vi "Main.vi"() -> ()   [LabVIEW 2021] (continued)
                    w601 = T9 9 items=["刷新间隔", "波特率", "布尔1设置项", "布尔2设置项", "布尔3设置项", "布尔4设置项", "布尔5设置项", "布尔6设置项", "布尔7设置项", "布尔8设置项", "显控1设置", "显控2设置", "显控3设置", "显控4设置", "显控5设置", "显控6设置", "显控7设置", "显控8设置", "显控9设置", "显控10设置", "显控11设置", "显控12设置", "设控1设置", "设控2设置", "设控3设置", "设控4设置", "设控5设置", "设控6设置", "设控7设置", "设控8设置", "曲线1设置", "曲线2设置", "曲线3设置", "曲线4设置", "曲线5设置", "曲线6设置", "曲线7设置", "曲线8设置", "曲线9设置", "曲线10设置", "曲线11设置", "曲线12设置", "曲线13设置", "曲线14设置", "曲线15设置", "曲线16设置", "曲线17设置", "曲线18设置", "曲线19设置", "曲线20设置", "曲线21设置", "曲线22设置", "曲线23设置", "曲线24设置", "曲线25设置", "曲线26设置", "曲线27设置", "曲线28设置", "曲线29设置", "曲线30设置", "曲线31设置", "曲线32设置", "曲线33设置", "曲线34设置", "曲线35设置", "曲线36设置", "曲线37设置", "曲线38设置", "曲线39设置", "曲线40设置", "曲线41设置", "曲线42设置", "曲线43设置", "曲线44设置", "曲线45设置", "曲线46设置", "曲线47设置", "曲线48设置", "曲线49设置", "曲线50设置", "曲线51设置", "曲线52设置", "曲线53设置", "曲线54设置", "曲线55设置", "曲线56设置", "曲线57设置", "曲线58设置", "曲线59设置", "曲线60设置", "曲线61设置", "曲线62设置", "曲线63设置", "曲线64设置", "ID值", "数据模式"] ("DataInitDef")
                    n457 = property on="表格" class="Tbl (严格)"() -> ("Selection Start"=w609:T1)  [unwired: 2 in, 2 out]
                    n458 = Unbundle By Name(w609) -> ("Row"=w608:i32)
                    n459 = property on="表格" class="Tbl (严格)"() -> ("Value"=w610:string[][])  [unwired: 2 in, 2 out]
                    n460 = Number To Decimal String(number=w608) -> (decimal integer string=w611:string)  [unwired: 1 in]
                    n461 = Index Array(array=w610, index (row)=w608, index (col)=0 ("禁用的索引 (列)")) -> (element=w607:string)
                    n462 = String Subset(string=w607, length (rest)=10 ("长度（剩余）")) -> (substring=w606:string)  [unwired: 1 in]
                    n463 = invoke on="控件配置文件" class="Tbl (严格)" method="Set Cell Value"("X Index"=1 ("X索引"), "Y Index"=w601, "Value"=w611) -> ()  [unwired: 3 in, 6 out]
                    n464 = property on="布尔 8" class="Bool (严格)"("Caption.Text"=w606) -> ()  [unwired: 2 in, 2 out]
                    n465 = property on="布控8设置" class="Str"("Val(Sgnl)"=w606) -> ()  [unwired: 2 in, 2 out]
                    n466 = invoke on="控件配置文件" class="Tbl (严格)" method="Set Cell Value"("X Index"=0 ("X索引"), "Y Index"=w601, "Value"=w606) -> ()  [unwired: 3 in, 6 out]
                  }
                  frame "关联到显控1" {
                    w612 = T9 10 items=["刷新间隔", "波特率", "布尔1设置项", "布尔2设置项", "布尔3设置项", "布尔4设置项", "布尔5设置项", "布尔6设置项", "布尔7设置项", "布尔8设置项", "显控1设置", "显控2设置", "显控3设置", "显控4设置", "显控5设置", "显控6设置", "显控7设置", "显控8设置", "显控9设置", "显控10设置", "显控11设置", "显控12设置", "设控1设置", "设控2设置", "设控3设置", "设控4设置", "设控5设置", "设控6设置", "设控7设置", "设控8设置", "曲线1设置", "曲线2设置", "曲线3设置", "曲线4设置", "曲线5设置", "曲线6设置", "曲线7设置", "曲线8设置", "曲线9设置", "曲线10设置", "曲线11设置", "曲线12设置", "曲线13设置", "曲线14设置", "曲线15设置", "曲线16设置", "曲线17设置", "曲线18设置", "曲线19设置", "曲线20设置", "曲线21设置", "曲线22设置", "曲线23设置", "曲线24设置", "曲线25设置", "曲线26设置", "曲线27设置", "曲线28设置", "曲线29设置", "曲线30设置", "曲线31设置", "曲线32设置", "曲线33设置", "曲线34设置", "曲线35设置", "曲线36设置", "曲线37设置", "曲线38设置", "曲线39设置", "曲线40设置", "曲线41设置", "曲线42设置", "曲线43设置", "曲线44设置", "曲线45设置", "曲线46设置", "曲线47设置", "曲线48设置", "曲线49设置", "曲线50设置", "曲线51设置", "曲线52设置", "曲线53设置", "曲线54设置", "曲线55设置", "曲线56设置", "曲线57设置", "曲线58设置", "曲线59设置", "曲线60设置", "曲线61设置", "曲线62设置", "曲线63设置", "曲线64设置", "ID值", "数据模式"] ("DataInitDef")
                    n467 = property on="表格" class="Tbl (严格)"() -> ("Selection Start"=w622:T1)  [unwired: 2 in, 2 out]
                    n468 = Unbundle By Name(w622) -> ("Row"=w619:i32)
                    n469 = property on="表格" class="Tbl (严格)"() -> ("Value"=w621:string[][])  [unwired: 2 in, 2 out]
                    n470 = Number To Decimal String(number=w619) -> (decimal integer string=w616:string)  [unwired: 1 in]
                    n471 = Index Array(array=w621, index (row)=w619, index (col)=0 ("禁用的索引 (列)")) -> (element=w614:string)
                    n472 = String Subset(string=w614, length (rest)=16 ("长度（剩余）")) -> (substring=w613:string)  [unwired: 1 in]
                    n473 = invoke on="控件配置文件" class="Tbl (严格)" method="Set Cell Value"("X Index"=1 ("X索引"), "Y Index"=w612, "Value"=w616) -> ()  [unwired: 3 in, 6 out]
                    n474 = property on="显控1设置" class="Str"("Val(Sgnl)"=w613) -> ()  [unwired: 2 in, 2 out]
                    n475 = property on="显控1" class="Str"("Caption.Text"=w613) -> ()  [unwired: 2 in, 2 out]
                    n476 = invoke on="控件配置文件" class="Tbl (严格)" method="Set Cell Value"("X Index"=0 ("X索引"), "Y Index"=w612, "Value"=w613) -> ()  [unwired: 3 in, 6 out]
                  }
                  frame "关联到显控2" {
                    w623 = T9 11 items=["刷新间隔", "波特率", "布尔1设置项", "布尔2设置项", "布尔3设置项", "布尔4设置项", "布尔5设置项", "布尔6设置项", "布尔7设置项", "布尔8设置项", "显控1设置", "显控2设置", "显控3设置", "显控4设置", "显控5设置", "显控6设置", "显控7设置", "显控8设置", "显控9设置", "显控10设置", "显控11设置", "显控12设置", "设控1设置", "设控2设置", "设控3设置", "设控4设置", "设控5设置", "设控6设置", "设控7设置", "设控8设置", "曲线1设置", "曲线2设置", "曲线3设置", "曲线4设置", "曲线5设置", "曲线6设置", "曲线7设置", "曲线8设置", "曲线9设置", "曲线10设置", "曲线11设置", "曲线12设置", "曲线13设置", "曲线14设置", "曲线15设置", "曲线16设置", "曲线17设置", "曲线18设置", "曲线19设置", "曲线20设置", "曲线21设置", "曲线22设置", "曲线23设置", "曲线24设置", "曲线25设置", "曲线26设置", "曲线27设置", "曲线28设置", "曲线29设置", "曲线30设置", "曲线31设置", "曲线32设置", "曲线33设置", "曲线34设置", "曲线35设置", "曲线36设置", "曲线37设置", "曲线38设置", "曲线39设置", "曲线40设置", "曲线41设置", "曲线42设置", "曲线43设置", "曲线44设置", "曲线45设置", "曲线46设置", "曲线47设置", "曲线48设置", "曲线49设置", "曲线50设置", "曲线51设置", "曲线52设置", "曲线53设置", "曲线54设置", "曲线55设置", "曲线56设置", "曲线57设置", "曲线58设置", "曲线59设置", "曲线60设置", "曲线61设置", "曲线62设置", "曲线63设置", "曲线64设置", "ID值", "数据模式"] ("DataInitDef")
                    n477 = property on="表格" class="Tbl (严格)"() -> ("Selection Start"=w632:T1)  [unwired: 2 in, 2 out]
                    n478 = Unbundle By Name(w632) -> ("Row"=w630:i32)
                    n479 = property on="表格" class="Tbl (严格)"() -> ("Value"=w631:string[][])  [unwired: 2 in, 2 out]
                    n480 = Number To Decimal String(number=w630) -> (decimal integer string=w627:string)  [unwired: 1 in]
                    n481 = Index Array(array=w631, index (row)=w630, index (col)=0 ("禁用的索引 (列)")) -> (element=w625:string)
                    n482 = String Subset(string=w625, length (rest)=16 ("长度（剩余）")) -> (substring=w624:string)  [unwired: 1 in]
                    n483 = invoke on="控件配置文件" class="Tbl (严格)" method="Set Cell Value"("X Index"=1 ("X索引"), "Y Index"=w623, "Value"=w627) -> ()  [unwired: 3 in, 6 out]
                    n484 = property on="显控2设置" class="Str"("Val(Sgnl)"=w624) -> ()  [unwired: 2 in, 2 out]
                    n485 = property on="显控2" class="Str"("Caption.Text"=w624) -> ()  [unwired: 2 in, 2 out]
                    n486 = invoke on="控件配置文件" class="Tbl (严格)" method="Set Cell Value"("X Index"=0 ("X索引"), "Y Index"=w623, "Value"=w624) -> ()  [unwired: 3 in, 6 out]
                  }
                  frame "关联到显控3" {
                    w634 = T9 12 items=["刷新间隔", "波特率", "布尔1设置项", "布尔2设置项", "布尔3设置项", "布尔4设置项", "布尔5设置项", "布尔6设置项", "布尔7设置项", "布尔8设置项", "显控1设置", "显控2设置", "显控3设置", "显控4设置", "显控5设置", "显控6设置", "显控7设置", "显控8设置", "显控9设置", "显控10设置", "显控11设置", "显控12设置", "设控1设置", "设控2设置", "设控3设置", "设控4设置", "设控5设置", "设控6设置", "设控7设置", "设控8设置", "曲线1设置", "曲线2设置", "曲线3设置", "曲线4设置", "曲线5设置", "曲线6设置", "曲线7设置", "曲线8设置", "曲线9设置", "曲线10设置", "曲线11设置", "曲线12设置", "曲线13设置", "曲线14设置", "曲线15设置", "曲线16设置", "曲线17设置", "曲线18设置", "曲线19设置", "曲线20设置", "曲线21设置", "曲线22设置", "曲线23设置", "曲线24设置", "曲线25设置", "曲线26设置", "曲线27设置", "曲线28设置", "曲线29设置", "曲线30设置", "曲线31设置", "曲线32设置", "曲线33设置", "曲线34设置", "曲线35设置", "曲线36设置", "曲线37设置", "曲线38设置", "曲线39设置", "曲线40设置", "曲线41设置", "曲线42设置", "曲线43设置", "曲线44设置", "曲线45设置", "曲线46设置", "曲线47设置", "曲线48设置", "曲线49设置", "曲线50设置", "曲线51设置", "曲线52设置", "曲线53设置", "曲线54设置", "曲线55设置", "曲线56设置", "曲线57设置", "曲线58设置", "曲线59设置", "曲线60设置", "曲线61设置", "曲线62设置", "曲线63设置", "曲线64设置", "ID值", "数据模式"] ("DataInitDef")
                    n487 = property on="表格" class="Tbl (严格)"() -> ("Selection Start"=w643:T1)  [unwired: 2 in, 2 out]
                    n488 = Unbundle By Name(w643) -> ("Row"=w641:i32)
                    n489 = property on="表格" class="Tbl (严格)"() -> ("Value"=w642:string[][])  [unwired: 2 in, 2 out]
                    n490 = Number To Decimal String(number=w641) -> (decimal integer string=w638:string)  [unwired: 1 in]
                    n491 = Index Array(array=w642, index (row)=w641, index (col)=0 ("禁用的索引 (列)")) -> (element=w636:string)
                    n492 = String Subset(string=w636, length (rest)=16 ("长度（剩余）")) -> (substring=w635:string)  [unwired: 1 in]
                    n493 = invoke on="控件配置文件" class="Tbl (严格)" method="Set Cell Value"("X Index"=1 ("X索引"), "Y Index"=w634, "Value"=w638) -> ()  [unwired: 3 in, 6 out]
                    n494 = property on="显控3设置" class="Str"("Val(Sgnl)"=w635) -> ()  [unwired: 2 in, 2 out]
                    n495 = property on="显控3" class="Str"("Caption.Text"=w635) -> ()  [unwired: 2 in, 2 out]
                    n496 = invoke on="控件配置文件" class="Tbl (严格)" method="Set Cell Value"("X Index"=0 ("X索引"), "Y Index"=w634, "Value"=w635) -> ()  [unwired: 3 in, 6 out]
                  }
                  frame "关联到显控4" {
                    w645 = T9 13 items=["刷新间隔", "波特率", "布尔1设置项", "布尔2设置项", "布尔3设置项", "布尔4设置项", "布尔5设置项", "布尔6设置项", "布尔7设置项", "布尔8设置项", "显控1设置", "显控2设置", "显控3设置", "显控4设置", "显控5设置", "显控6设置", "显控7设置", "显控8设置", "显控9设置", "显控10设置", "显控11设置", "显控12设置", "设控1设置", "设控2设置", "设控3设置", "设控4设置", "设控5设置", "设控6设置", "设控7设置", "设控8设置", "曲线1设置", "曲线2设置", "曲线3设置", "曲线4设置", "曲线5设置", "曲线6设置", "曲线7设置", "曲线8设置", "曲线9设置", "曲线10设置", "曲线11设置", "曲线12设置", "曲线13设置", "曲线14设置", "曲线15设置", "曲线16设置", "曲线17设置", "曲线18设置", "曲线19设置", "曲线20设置", "曲线21设置", "曲线22设置", "曲线23设置", "曲线24设置", "曲线25设置", "曲线26设置", "曲线27设置", "曲线28设置", "曲线29设置", "曲线30设置", "曲线31设置", "曲线32设置", "曲线33设置", "曲线34设置", "曲线35设置", "曲线36设置", "曲线37设置", "曲线38设置", "曲线39设置", "曲线40设置", "曲线41设置", "曲线42设置", "曲线43设置", "曲线44设置", "曲线45设置", "曲线46设置", "曲线47设置", "曲线48设置", "曲线49设置", "曲线50设置", "曲线51设置", "曲线52设置", "曲线53设置", "曲线54设置", "曲线55设置", "曲线56设置", "曲线57设置", "曲线58设置", "曲线59设置", "曲线60设置", "曲线61设置", "曲线62设置", "曲线63设置", "曲线64设置", "ID值", "数据模式"] ("DataInitDef")
                    n497 = property on="表格" class="Tbl (严格)"() -> ("Selection Start"=w654:T1)  [unwired: 2 in, 2 out]
                    n498 = Unbundle By Name(w654) -> ("Row"=w652:i32)
                    n499 = property on="表格" class="Tbl (严格)"() -> ("Value"=w653:string[][])  [unwired: 2 in, 2 out]
                    n500 = Number To Decimal String(number=w652) -> (decimal integer string=w649:string)  [unwired: 1 in]
                    n501 = Index Array(array=w653, index (row)=w652, index (col)=0 ("禁用的索引 (列)")) -> (element=w647:string)
                    n502 = String Subset(string=w647, length (rest)=16 ("长度（剩余）")) -> (substring=w646:string)  [unwired: 1 in]
                    n503 = invoke on="控件配置文件" class="Tbl (严格)" method="Set Cell Value"("X Index"=1 ("X索引"), "Y Index"=w645, "Value"=w649) -> ()  [unwired: 3 in, 6 out]
                    n504 = property on="显控4设置" class="Str"("Val(Sgnl)"=w646) -> ()  [unwired: 2 in, 2 out]
                    n505 = property on="显控4" class="Str"("Caption.Text"=w646) -> ()  [unwired: 2 in, 2 out]
                    n506 = invoke on="控件配置文件" class="Tbl (严格)" method="Set Cell Value"("X Index"=0 ("X索引"), "Y Index"=w645, "Value"=w646) -> ()  [unwired: 3 in, 6 out]
                  }
                  frame "关联到显控5" {
                    w656 = T9 14 items=["刷新间隔", "波特率", "布尔1设置项", "布尔2设置项", "布尔3设置项", "布尔4设置项", "布尔5设置项", "布尔6设置项", "布尔7设置项", "布尔8设置项", "显控1设置", "显控2设置", "显控3设置", "显控4设置", "显控5设置", "显控6设置", "显控7设置", "显控8设置", "显控9设置", "显控10设置", "显控11设置", "显控12设置", "设控1设置", "设控2设置", "设控3设置", "设控4设置", "设控5设置", "设控6设置", "设控7设置", "设控8设置", "曲线1设置", "曲线2设置", "曲线3设置", "曲线4设置", "曲线5设置", "曲线6设置", "曲线7设置", "曲线8设置", "曲线9设置", "曲线10设置", "曲线11设置", "曲线12设置", "曲线13设置", "曲线14设置", "曲线15设置", "曲线16设置", "曲线17设置", "曲线18设置", "曲线19设置", "曲线20设置", "曲线21设置", "曲线22设置", "曲线23设置", "曲线24设置", "曲线25设置", "曲线26设置", "曲线27设置", "曲线28设置", "曲线29设置", "曲线30设置", "曲线31设置", "曲线32设置", "曲线33设置", "曲线34设置", "曲线35设置", "曲线36设置", "曲线37设置", "曲线38设置", "曲线39设置", "曲线40设置", "曲线41设置", "曲线42设置", "曲线43设置", "曲线44设置", "曲线45设置", "曲线46设置", "曲线47设置", "曲线48设置", "曲线49设置", "曲线50设置", "曲线51设置", "曲线52设置", "曲线53设置", "曲线54设置", "曲线55设置", "曲线56设置", "曲线57设置", "曲线58设置", "曲线59设置", "曲线60设置", "曲线61设置", "曲线62设置", "曲线63设置", "曲线64设置", "ID值", "数据模式"] ("DataInitDef")
                    n507 = property on="表格" class="Tbl (严格)"() -> ("Selection Start"=w665:T1)  [unwired: 2 in, 2 out]
                    n508 = Unbundle By Name(w665) -> ("Row"=w663:i32)
                    n509 = property on="表格" class="Tbl (严格)"() -> ("Value"=w664:string[][])  [unwired: 2 in, 2 out]
                    n510 = Number To Decimal String(number=w663) -> (decimal integer string=w660:string)  [unwired: 1 in]
                    n511 = Index Array(array=w664, index (row)=w663, index (col)=0 ("禁用的索引 (列)")) -> (element=w658:string)
                    n512 = String Subset(string=w658, length (rest)=16 ("长度（剩余）")) -> (substring=w657:string)  [unwired: 1 in]
                    n513 = invoke on="控件配置文件" class="Tbl (严格)" method="Set Cell Value"("X Index"=1 ("X索引"), "Y Index"=w656, "Value"=w660) -> ()  [unwired: 3 in, 6 out]
                    n514 = property on="显控5设置" class="Str"("Val(Sgnl)"=w657) -> ()  [unwired: 2 in, 2 out]
                    n515 = property on="显控5" class="Str"("Caption.Text"=w657) -> ()  [unwired: 2 in, 2 out]
                    n516 = invoke on="控件配置文件" class="Tbl (严格)" method="Set Cell Value"("X Index"=0 ("X索引"), "Y Index"=w656, "Value"=w657) -> ()  [unwired: 3 in, 6 out]
                  }
                  frame "关联到显控6" {
                    w667 = T9 15 items=["刷新间隔", "波特率", "布尔1设置项", "布尔2设置项", "布尔3设置项", "布尔4设置项", "布尔5设置项", "布尔6设置项", "布尔7设置项", "布尔8设置项", "显控1设置", "显控2设置", "显控3设置", "显控4设置", "显控5设置", "显控6设置", "显控7设置", "显控8设置", "显控9设置", "显控10设置", "显控11设置", "显控12设置", "设控1设置", "设控2设置", "设控3设置", "设控4设置", "设控5设置", "设控6设置", "设控7设置", "设控8设置", "曲线1设置", "曲线2设置", "曲线3设置", "曲线4设置", "曲线5设置", "曲线6设置", "曲线7设置", "曲线8设置", "曲线9设置", "曲线10设置", "曲线11设置", "曲线12设置", "曲线13设置", "曲线14设置", "曲线15设置", "曲线16设置", "曲线17设置", "曲线18设置", "曲线19设置", "曲线20设置", "曲线21设置", "曲线22设置", "曲线23设置", "曲线24设置", "曲线25设置", "曲线26设置", "曲线27设置", "曲线28设置", "曲线29设置", "曲线30设置", "曲线31设置", "曲线32设置", "曲线33设置", "曲线34设置", "曲线35设置", "曲线36设置", "曲线37设置", "曲线38设置", "曲线39设置", "曲线40设置", "曲线41设置", "曲线42设置", "曲线43设置", "曲线44设置", "曲线45设置", "曲线46设置", "曲线47设置", "曲线48设置", "曲线49设置", "曲线50设置", "曲线51设置", "曲线52设置", "曲线53设置", "曲线54设置", "曲线55设置", "曲线56设置", "曲线57设置", "曲线58设置", "曲线59设置", "曲线60设置", "曲线61设置", "曲线62设置", "曲线63设置", "曲线64设置", "ID值", "数据模式"] ("DataInitDef")
                    n517 = property on="表格" class="Tbl (严格)"() -> ("Selection Start"=w676:T1)  [unwired: 2 in, 2 out]
                    n518 = Unbundle By Name(w676) -> ("Row"=w674:i32)
                    n519 = property on="表格" class="Tbl (严格)"() -> ("Value"=w675:string[][])  [unwired: 2 in, 2 out]
                    n520 = Number To Decimal String(number=w674) -> (decimal integer string=w671:string)  [unwired: 1 in]
                    n521 = Index Array(array=w675, index (row)=w674, index (col)=0 ("禁用的索引 (列)")) -> (element=w669:string)
                    n522 = String Subset(string=w669, length (rest)=16 ("长度（剩余）")) -> (substring=w668:string)  [unwired: 1 in]
                    n523 = invoke on="控件配置文件" class="Tbl (严格)" method="Set Cell Value"("X Index"=1 ("X索引"), "Y Index"=w667, "Value"=w671) -> ()  [unwired: 3 in, 6 out]
                    n524 = property on="显控6设置" class="Str"("Val(Sgnl)"=w668) -> ()  [unwired: 2 in, 2 out]
                    n525 = property on="显控6" class="Str"("Caption.Text"=w668) -> ()  [unwired: 2 in, 2 out]
                    n526 = invoke on="控件配置文件" class="Tbl (严格)" method="Set Cell Value"("X Index"=0 ("X索引"), "Y Index"=w667, "Value"=w668) -> ()  [unwired: 3 in, 6 out]
                  }
                  frame "关联到显控7" {
                    w678 = T9 16 items=["刷新间隔", "波特率", "布尔1设置项", "布尔2设置项", "布尔3设置项", "布尔4设置项", "布尔5设置项", "布尔6设置项", "布尔7设置项", "布尔8设置项", "显控1设置", "显控2设置", "显控3设置", "显控4设置", "显控5设置", "显控6设置", "显控7设置", "显控8设置", "显控9设置", "显控10设置", "显控11设置", "显控12设置", "设控1设置", "设控2设置", "设控3设置", "设控4设置", "设控5设置", "设控6设置", "设控7设置", "设控8设置", "曲线1设置", "曲线2设置", "曲线3设置", "曲线4设置", "曲线5设置", "曲线6设置", "曲线7设置", "曲线8设置", "曲线9设置", "曲线10设置", "曲线11设置", "曲线12设置", "曲线13设置", "曲线14设置", "曲线15设置", "曲线16设置", "曲线17设置", "曲线18设置", "曲线19设置", "曲线20设置", "曲线21设置", "曲线22设置", "曲线23设置", "曲线24设置", "曲线25设置", "曲线26设置", "曲线27设置", "曲线28设置", "曲线29设置", "曲线30设置", "曲线31设置", "曲线32设置", "曲线33设置", "曲线34设置", "曲线35设置", "曲线36设置", "曲线37设置", "曲线38设置", "曲线39设置", "曲线40设置", "曲线41设置", "曲线42设置", "曲线43设置", "曲线44设置", "曲线45设置", "曲线46设置", "曲线47设置", "曲线48设置", "曲线49设置", "曲线50设置", "曲线51设置", "曲线52设置", "曲线53设置", "曲线54设置", "曲线55设置", "曲线56设置", "曲线57设置", "曲线58设置", "曲线59设置", "曲线60设置", "曲线61设置", "曲线62设置", "曲线63设置", "曲线64设置", "ID值", "数据模式"] ("DataInitDef")
                    n527 = property on="表格" class="Tbl (严格)"() -> ("Selection Start"=w687:T1)  [unwired: 2 in, 2 out]
                    n528 = Unbundle By Name(w687) -> ("Row"=w685:i32)
                    n529 = property on="表格" class="Tbl (严格)"() -> ("Value"=w686:string[][])  [unwired: 2 in, 2 out]
                    n530 = Number To Decimal String(number=w685) -> (decimal integer string=w682:string)  [unwired: 1 in]
                    n531 = Index Array(array=w686, index (row)=w685, index (col)=0 ("禁用的索引 (列)")) -> (element=w680:string)
                    n532 = String Subset(string=w680, length (rest)=16 ("长度（剩余）")) -> (substring=w679:string)  [unwired: 1 in]
                    n533 = invoke on="控件配置文件" class="Tbl (严格)" method="Set Cell Value"("X Index"=1 ("X索引"), "Y Index"=w678, "Value"=w682) -> ()  [unwired: 3 in, 6 out]
                    n534 = property on="显控7设置" class="Str"("Val(Sgnl)"=w679) -> ()  [unwired: 2 in, 2 out]
                    n535 = property on="显控7" class="Str"("Caption.Text"=w679) -> ()  [unwired: 2 in, 2 out]
                    n536 = invoke on="控件配置文件" class="Tbl (严格)" method="Set Cell Value"("X Index"=0 ("X索引"), "Y Index"=w678, "Value"=w679) -> ()  [unwired: 3 in, 6 out]
                  }
                  frame "关联到显控8" {
                    w689 = T9 17 items=["刷新间隔", "波特率", "布尔1设置项", "布尔2设置项", "布尔3设置项", "布尔4设置项", "布尔5设置项", "布尔6设置项", "布尔7设置项", "布尔8设置项", "显控1设置", "显控2设置", "显控3设置", "显控4设置", "显控5设置", "显控6设置", "显控7设置", "显控8设置", "显控9设置", "显控10设置", "显控11设置", "显控12设置", "设控1设置", "设控2设置", "设控3设置", "设控4设置", "设控5设置", "设控6设置", "设控7设置", "设控8设置", "曲线1设置", "曲线2设置", "曲线3设置", "曲线4设置", "曲线5设置", "曲线6设置", "曲线7设置", "曲线8设置", "曲线9设置", "曲线10设置", "曲线11设置", "曲线12设置", "曲线13设置", "曲线14设置", "曲线15设置", "曲线16设置", "曲线17设置", "曲线18设置", "曲线19设置", "曲线20设置", "曲线21设置", "曲线22设置", "曲线23设置", "曲线24设置", "曲线25设置", "曲线26设置", "曲线27设置", "曲线28设置", "曲线29设置", "曲线30设置", "曲线31设置", "曲线32设置", "曲线33设置", "曲线34设置", "曲线35设置", "曲线36设置", "曲线37设置", "曲线38设置", "曲线39设置", "曲线40设置", "曲线41设置", "曲线42设置", "曲线43设置", "曲线44设置", "曲线45设置", "曲线46设置", "曲线47设置", "曲线48设置", "曲线49设置", "曲线50设置", "曲线51设置", "曲线52设置", "曲线53设置", "曲线54设置", "曲线55设置", "曲线56设置", "曲线57设置", "曲线58设置", "曲线59设置", "曲线60设置", "曲线61设置", "曲线62设置", "曲线63设置", "曲线64设置", "ID值", "数据模式"] ("DataInitDef")
                    n537 = property on="表格" class="Tbl (严格)"() -> ("Selection Start"=w698:T1)  [unwired: 2 in, 2 out]
                    n538 = Unbundle By Name(w698) -> ("Row"=w696:i32)
                    n539 = property on="表格" class="Tbl (严格)"() -> ("Value"=w697:string[][])  [unwired: 2 in, 2 out]
                    n540 = Number To Decimal String(number=w696) -> (decimal integer string=w693:string)  [unwired: 1 in]
                    n541 = Index Array(array=w697, index (row)=w696, index (col)=0 ("禁用的索引 (列)")) -> (element=w691:string)
                    n542 = String Subset(string=w691, length (rest)=16 ("长度（剩余）")) -> (substring=w690:string)  [unwired: 1 in]
                    n543 = invoke on="控件配置文件" class="Tbl (严格)" method="Set Cell Value"("X Index"=1 ("X索引"), "Y Index"=w689, "Value"=w693) -> ()  [unwired: 3 in, 6 out]
                    n544 = property on="显控8设置" class="Str"("Val(Sgnl)"=w690) -> ()  [unwired: 2 in, 2 out]
                    n545 = property on="显控8" class="Str"("Caption.Text"=w690) -> ()  [unwired: 2 in, 2 out]
                    n546 = invoke on="控件配置文件" class="Tbl (严格)" method="Set Cell Value"("X Index"=0 ("X索引"), "Y Index"=w689, "Value"=w690) -> ()  [unwired: 3 in, 6 out]
                  }
                  frame "关联到显控9" {
                    w700 = T9 18 items=["刷新间隔", "波特率", "布尔1设置项", "布尔2设置项", "布尔3设置项", "布尔4设置项", "布尔5设置项", "布尔6设置项", "布尔7设置项", "布尔8设置项", "显控1设置", "显控2设置", "显控3设置", "显控4设置", "显控5设置", "显控6设置", "显控7设置", "显控8设置", "显控9设置", "显控10设置", "显控11设置", "显控12设置", "设控1设置", "设控2设置", "设控3设置", "设控4设置", "设控5设置", "设控6设置", "设控7设置", "设控8设置", "曲线1设置", "曲线2设置", "曲线3设置", "曲线4设置", "曲线5设置", "曲线6设置", "曲线7设置", "曲线8设置", "曲线9设置", "曲线10设置", "曲线11设置", "曲线12设置", "曲线13设置", "曲线14设置", "曲线15设置", "曲线16设置", "曲线17设置", "曲线18设置", "曲线19设置", "曲线20设置", "曲线21设置", "曲线22设置", "曲线23设置", "曲线24设置", "曲线25设置", "曲线26设置", "曲线27设置", "曲线28设置", "曲线29设置", "曲线30设置", "曲线31设置", "曲线32设置", "曲线33设置", "曲线34设置", "曲线35设置", "曲线36设置", "曲线37设置", "曲线38设置", "曲线39设置", "曲线40设置", "曲线41设置", "曲线42设置", "曲线43设置", "曲线44设置", "曲线45设置", "曲线46设置", "曲线47设置", "曲线48设置", "曲线49设置", "曲线50设置", "曲线51设置", "曲线52设置", "曲线53设置", "曲线54设置", "曲线55设置", "曲线56设置", "曲线57设置", "曲线58设置", "曲线59设置", "曲线60设置", "曲线61设置", "曲线62设置", "曲线63设置", "曲线64设置", "ID值", "数据模式"] ("DataInitDef")
                    n547 = property on="表格" class="Tbl (严格)"() -> ("Selection Start"=w709:T1)  [unwired: 2 in, 2 out]
                    n548 = Unbundle By Name(w709) -> ("Row"=w707:i32)
                    n549 = property on="表格" class="Tbl (严格)"() -> ("Value"=w708:string[][])  [unwired: 2 in, 2 out]
                    n550 = Number To Decimal String(number=w707) -> (decimal integer string=w704:string)  [unwired: 1 in]
                    n551 = Index Array(array=w708, index (row)=w707, index (col)=0 ("禁用的索引 (列)")) -> (element=w702:string)
                    n552 = String Subset(string=w702, length (rest)=16 ("长度（剩余）")) -> (substring=w701:string)  [unwired: 1 in]
                    n553 = invoke on="控件配置文件" class="Tbl (严格)" method="Set Cell Value"("X Index"=1 ("X索引"), "Y Index"=w700, "Value"=w704) -> ()  [unwired: 3 in, 6 out]
                    n554 = property on="显控9设置" class="Str"("Val(Sgnl)"=w701) -> ()  [unwired: 2 in, 2 out]
                    n555 = property on="显控9" class="Str"("Caption.Text"=w701) -> ()  [unwired: 2 in, 2 out]
                    n556 = invoke on="控件配置文件" class="Tbl (严格)" method="Set Cell Value"("X Index"=0 ("X索引"), "Y Index"=w700, "Value"=w701) -> ()  [unwired: 3 in, 6 out]
                  }
                  frame "关联到显控10" {
                    w711 = T9 19 items=["刷新间隔", "波特率", "布尔1设置项", "布尔2设置项", "布尔3设置项", "布尔4设置项", "布尔5设置项", "布尔6设置项", "布尔7设置项", "布尔8设置项", "显控1设置", "显控2设置", "显控3设置", "显控4设置", "显控5设置", "显控6设置", "显控7设置", "显控8设置", "显控9设置", "显控10设置", "显控11设置", "显控12设置", "设控1设置", "设控2设置", "设控3设置", "设控4设置", "设控5设置", "设控6设置", "设控7设置", "设控8设置", "曲线1设置", "曲线2设置", "曲线3设置", "曲线4设置", "曲线5设置", "曲线6设置", "曲线7设置", "曲线8设置", "曲线9设置", "曲线10设置", "曲线11设置", "曲线12设置", "曲线13设置", "曲线14设置", "曲线15设置", "曲线16设置", "曲线17设置", "曲线18设置", "曲线19设置", "曲线20设置", "曲线21设置", "曲线22设置", "曲线23设置", "曲线24设置", "曲线25设置", "曲线26设置", "曲线27设置", "曲线28设置", "曲线29设置", "曲线30设置", "曲线31设置", "曲线32设置", "曲线33设置", "曲线34设置", "曲线35设置", "曲线36设置", "曲线37设置", "曲线38设置", "曲线39设置", "曲线40设置", "曲线41设置", "曲线42设置", "曲线43设置", "曲线44设置", "曲线45设置", "曲线46设置", "曲线47设置", "曲线48设置", "曲线49设置", "曲线50设置", "曲线51设置", "曲线52设置", "曲线53设置", "曲线54设置", "曲线55设置", "曲线56设置", "曲线57设置", "曲线58设置", "曲线59设置", "曲线60设置", "曲线61设置", "曲线62设置", "曲线63设置", "曲线64设置", "ID值", "数据模式"] ("DataInitDef")
                    n557 = property on="表格" class="Tbl (严格)"() -> ("Selection Start"=w720:T1)  [unwired: 2 in, 2 out]
                    n558 = Unbundle By Name(w720) -> ("Row"=w718:i32)
                    n559 = property on="表格" class="Tbl (严格)"() -> ("Value"=w719:string[][])  [unwired: 2 in, 2 out]
                    n560 = Number To Decimal String(number=w718) -> (decimal integer string=w715:string)  [unwired: 1 in]
                    n561 = Index Array(array=w719, index (row)=w718, index (col)=0 ("禁用的索引 (列)")) -> (element=w713:string)
                    n562 = String Subset(string=w713, length (rest)=16 ("长度（剩余）")) -> (substring=w712:string)  [unwired: 1 in]
                    n563 = invoke on="控件配置文件" class="Tbl (严格)" method="Set Cell Value"("X Index"=1 ("X索引"), "Y Index"=w711, "Value"=w715) -> ()  [unwired: 3 in, 6 out]
                    n564 = property on="显控10" class="Str"("Caption.Text"=w712) -> ()  [unwired: 2 in, 2 out]
                    n565 = property on="显控10设置" class="Str"("Val(Sgnl)"=w712) -> ()  [unwired: 2 in, 2 out]
                    n566 = invoke on="控件配置文件" class="Tbl (严格)" method="Set Cell Value"("X Index"=0 ("X索引"), "Y Index"=w711, "Value"=w712) -> ()  [unwired: 3 in, 6 out]
                  }
                  frame "关联到显控11" {
                    w722 = T9 20 items=["刷新间隔", "波特率", "布尔1设置项", "布尔2设置项", "布尔3设置项", "布尔4设置项", "布尔5设置项", "布尔6设置项", "布尔7设置项", "布尔8设置项", "显控1设置", "显控2设置", "显控3设置", "显控4设置", "显控5设置", "显控6设置", "显控7设置", "显控8设置", "显控9设置", "显控10设置", "显控11设置", "显控12设置", "设控1设置", "设控2设置", "设控3设置", "设控4设置", "设控5设置", "设控6设置", "设控7设置", "设控8设置", "曲线1设置", "曲线2设置", "曲线3设置", "曲线4设置", "曲线5设置", "曲线6设置", "曲线7设置", "曲线8设置", "曲线9设置", "曲线10设置", "曲线11设置", "曲线12设置", "曲线13设置", "曲线14设置", "曲线15设置", "曲线16设置", "曲线17设置", "曲线18设置", "曲线19设置", "曲线20设置", "曲线21设置", "曲线22设置", "曲线23设置", "曲线24设置", "曲线25设置", "曲线26设置", "曲线27设置", "曲线28设置", "曲线29设置", "曲线30设置", "曲线31设置", "曲线32设置", "曲线33设置", "曲线34设置", "曲线35设置", "曲线36设置", "曲线37设置", "曲线38设置", "曲线39设置", "曲线40设置", "曲线41设置", "曲线42设置", "曲线43设置", "曲线44设置", "曲线45设置", "曲线46设置", "曲线47设置", "曲线48设置", "曲线49设置", "曲线50设置", "曲线51设置", "曲线52设置", "曲线53设置", "曲线54设置", "曲线55设置", "曲线56设置", "曲线57设置", "曲线58设置", "曲线59设置", "曲线60设置", "曲线61设置", "曲线62设置", "曲线63设置", "曲线64设置", "ID值", "数据模式"] ("DataInitDef")
                    n567 = property on="表格" class="Tbl (严格)"() -> ("Selection Start"=w731:T1)  [unwired: 2 in, 2 out]
                    n568 = Unbundle By Name(w731) -> ("Row"=w729:i32)
                    n569 = property on="表格" class="Tbl (严格)"() -> ("Value"=w730:string[][])  [unwired: 2 in, 2 out]
                    n570 = Number To Decimal String(number=w729) -> (decimal integer string=w726:string)  [unwired: 1 in]
                    n571 = Index Array(array=w730, index (row)=w729, index (col)=0 ("禁用的索引 (列)")) -> (element=w724:string)
                    n572 = String Subset(string=w724, length (rest)=16 ("长度（剩余）")) -> (substring=w723:string)  [unwired: 1 in]
                    n573 = invoke on="控件配置文件" class="Tbl (严格)" method="Set Cell Value"("X Index"=1 ("X索引"), "Y Index"=w722, "Value"=w726) -> ()  [unwired: 3 in, 6 out]
                    n574 = property on="显控11" class="Str"("Caption.Text"=w723) -> ()  [unwired: 2 in, 2 out]
                    n575 = property on="显控11设置" class="Str"("Val(Sgnl)"=w723) -> ()  [unwired: 2 in, 2 out]
                    n576 = invoke on="控件配置文件" class="Tbl (严格)" method="Set Cell Value"("X Index"=0 ("X索引"), "Y Index"=w722, "Value"=w723) -> ()  [unwired: 3 in, 6 out]
                  }
                  frame "关联到显控12" {
                    w733 = T9 21 items=["刷新间隔", "波特率", "布尔1设置项", "布尔2设置项", "布尔3设置项", "布尔4设置项", "布尔5设置项", "布尔6设置项", "布尔7设置项", "布尔8设置项", "显控1设置", "显控2设置", "显控3设置", "显控4设置", "显控5设置", "显控6设置", "显控7设置", "显控8设置", "显控9设置", "显控10设置", "显控11设置", "显控12设置", "设控1设置", "设控2设置", "设控3设置", "设控4设置", "设控5设置", "设控6设置", "设控7设置", "设控8设置", "曲线1设置", "曲线2设置", "曲线3设置", "曲线4设置", "曲线5设置", "曲线6设置", "曲线7设置", "曲线8设置", "曲线9设置", "曲线10设置", "曲线11设置", "曲线12设置", "曲线13设置", "曲线14设置", "曲线15设置", "曲线16设置", "曲线17设置", "曲线18设置", "曲线19设置", "曲线20设置", "曲线21设置", "曲线22设置", "曲线23设置", "曲线24设置", "曲线25设置", "曲线26设置", "曲线27设置", "曲线28设置", "曲线29设置", "曲线30设置", "曲线31设置", "曲线32设置", "曲线33设置", "曲线34设置", "曲线35设置", "曲线36设置", "曲线37设置", "曲线38设置", "曲线39设置", "曲线40设置", "曲线41设置", "曲线42设置", "曲线43设置", "曲线44设置", "曲线45设置", "曲线46设置", "曲线47设置", "曲线48设置", "曲线49设置", "曲线50设置", "曲线51设置", "曲线52设置", "曲线53设置", "曲线54设置", "曲线55设置", "曲线56设置", "曲线57设置", "曲线58设置", "曲线59设置", "曲线60设置", "曲线61设置", "曲线62设置", "曲线63设置", "曲线64设置", "ID值", "数据模式"] ("DataInitDef")
                    n577 = property on="表格" class="Tbl (严格)"() -> ("Selection Start"=w742:T1)  [unwired: 2 in, 2 out]
                    n578 = Unbundle By Name(w742) -> ("Row"=w740:i32)
                    n579 = property on="表格" class="Tbl (严格)"() -> ("Value"=w741:string[][])  [unwired: 2 in, 2 out]
                    n580 = Number To Decimal String(number=w740) -> (decimal integer string=w737:string)  [unwired: 1 in]
                    n581 = Index Array(array=w741, index (row)=w740, index (col)=0 ("禁用的索引 (列)")) -> (element=w735:string)
                    n582 = String Subset(string=w735, length (rest)=16 ("长度（剩余）")) -> (substring=w734:string)  [unwired: 1 in]
                    n583 = invoke on="控件配置文件" class="Tbl (严格)" method="Set Cell Value"("X Index"=1 ("X索引"), "Y Index"=w733, "Value"=w737) -> ()  [unwired: 3 in, 6 out]
                    n584 = property on="显控12" class="Str"("Caption.Text"=w734) -> ()  [unwired: 2 in, 2 out]
                    n585 = property on="显控12设置" class="Str"("Val(Sgnl)"=w734) -> ()  [unwired: 2 in, 2 out]
                    n586 = invoke on="控件配置文件" class="Tbl (严格)" method="Set Cell Value"("X Index"=0 ("X索引"), "Y Index"=w733, "Value"=w734) -> ()  [unwired: 3 in, 6 out]
                  }
                  frame "关联到曲线1" {
                    w744 = T9 30 items=["刷新间隔", "波特率", "布尔1设置项", "布尔2设置项", "布尔3设置项", "布尔4设置项", "布尔5设置项", "布尔6设置项", "布尔7设置项", "布尔8设置项", "显控1设置", "显控2设置", "显控3设置", "显控4设置", "显控5设置", "显控6设置", "显控7设置", "显控8设置", "显控9设置", "显控10设置", "显控11设置", "显控12设置", "设控1设置", "设控2设置", "设控3设置", "设控4设置", "设控5设置", "设控6设置", "设控7设置", "设控8设置", "曲线1设置", "曲线2设置", "曲线3设置", "曲线4设置", "曲线5设置", "曲线6设置", "曲线7设置", "曲线8设置", "曲线9设置", "曲线10设置", "曲线11设置", "曲线12设置", "曲线13设置", "曲线14设置", "曲线15设置", "曲线16设置", "曲线17设置", "曲线18设置", "曲线19设置", "曲线20设置", "曲线21设置", "曲线22设置", "曲线23设置", "曲线24设置", "曲线25设置", "曲线26设置", "曲线27设置", "曲线28设置", "曲线29设置", "曲线30设置", "曲线31设置", "曲线32设置", "曲线33设置", "曲线34设置", "曲线35设置", "曲线36设置", "曲线37设置", "曲线38设置", "曲线39设置", "曲线40设置", "曲线41设置", "曲线42设置", "曲线43设置", "曲线44设置", "曲线45设置", "曲线46设置", "曲线47设置", "曲线48设置", "曲线49设置", "曲线50设置", "曲线51设置", "曲线52设置", "曲线53设置", "曲线54设置", "曲线55设置", "曲线56设置", "曲线57设置", "曲线58设置", "曲线59设置", "曲线60设置", "曲线61设置", "曲线62设置", "曲线63设置", "曲线64设置", "ID值", "数据模式"] ("DataInitDef")
                    n587 = property on="表格" class="Tbl (严格)"() -> ("Selection Start"=w753:T1)  [unwired: 2 in, 2 out]
                    n588 = Unbundle By Name(w753) -> ("Row"=w751:i32)
                    n589 = property on="表格" class="Tbl (严格)"() -> ("Value"=w752:string[][])  [unwired: 2 in, 2 out]
                    n590 = Number To Decimal String(number=w751) -> (decimal integer string=w748:string)  [unwired: 1 in]
                    n591 = Index Array(array=w752, index (row)=w751, index (col)=0 ("禁用的索引 (列)")) -> (element=w746:string)
                    n592 = String Subset(string=w746, length (rest)=16 ("长度（剩余）")) -> (substring=w745:string)  [unwired: 1 in]
                    n593 = property on="曲线1设置" class="Str"("Val(Sgnl)"=w745) -> ()  [unwired: 2 in, 2 out]
                    n594 = invoke on="控件配置文件" class="Tbl (严格)" method="Set Cell Value"("X Index"=1 ("X索引"), "Y Index"=w744, "Value"=w748) -> ()  [unwired: 3 in, 6 out]
                    n595 = invoke on="控件配置文件" class="Tbl (严格)" method="Set Cell Value"("X Index"=0 ("X索引"), "Y Index"=w744, "Value"=w745) -> ()  [unwired: 3 in, 6 out]
                  }
                  frame "关联到曲线2" {
                    w755 = T9 31 items=["刷新间隔", "波特率", "布尔1设置项", "布尔2设置项", "布尔3设置项", "布尔4设置项", "布尔5设置项", "布尔6设置项", "布尔7设置项", "布尔8设置项", "显控1设置", "显控2设置", "显控3设置", "显控4设置", "显控5设置", "显控6设置", "显控7设置", "显控8设置", "显控9设置", "显控10设置", "显控11设置", "显控12设置", "设控1设置", "设控2设置", "设控3设置", "设控4设置", "设控5设置", "设控6设置", "设控7设置", "设控8设置", "曲线1设置", "曲线2设置", "曲线3设置", "曲线4设置", "曲线5设置", "曲线6设置", "曲线7设置", "曲线8设置", "曲线9设置", "曲线10设置", "曲线11设置", "曲线12设置", "曲线13设置", "曲线14设置", "曲线15设置", "曲线16设置", "曲线17设置", "曲线18设置", "曲线19设置", "曲线20设置", "曲线21设置", "曲线22设置", "曲线23设置", "曲线24设置", "曲线25设置", "曲线26设置", "曲线27设置", "曲线28设置", "曲线29设置", "曲线30设置", "曲线31设置", "曲线32设置", "曲线33设置", "曲线34设置", "曲线35设置", "曲线36设置", "曲线37设置", "曲线38设置", "曲线39设置", "曲线40设置", "曲线41设置", "曲线42设置", "曲线43设置", "曲线44设置", "曲线45设置", "曲线46设置", "曲线47设置", "曲线48设置", "曲线49设置", "曲线50设置", "曲线51设置", "曲线52设置", "曲线53设置", "曲线54设置", "曲线55设置", "曲线56设置", "曲线57设置", "曲线58设置", "曲线59设置", "曲线60设置", "曲线61设置", "曲线62设置", "曲线63设置", "曲线64设置", "ID值", "数据模式"] ("DataInitDef")
                    n596 = property on="表格" class="Tbl (严格)"() -> ("Selection Start"=w764:T1)  [unwired: 2 in, 2 out]
                    n597 = Unbundle By Name(w764) -> ("Row"=w762:i32)
                    n598 = property on="表格" class="Tbl (严格)"() -> ("Value"=w763:string[][])  [unwired: 2 in, 2 out]
                    n599 = Number To Decimal String(number=w762) -> (decimal integer string=w759:string)  [unwired: 1 in]
                    n600 = Index Array(array=w763, index (row)=w762, index (col)=0 ("禁用的索引 (列)")) -> (element=w757:string)
                    n601 = String Subset(string=w757, length (rest)=16 ("长度（剩余）")) -> (substring=w756:string)  [unwired: 1 in]
                    n602 = property on="曲线2设置" class="Str"("Val(Sgnl)"=w756) -> ()  [unwired: 2 in, 2 out]
                    n603 = invoke on="控件配置文件" class="Tbl (严格)" method="Set Cell Value"("X Index"=1 ("X索引"), "Y Index"=w755, "Value"=w759) -> ()  [unwired: 3 in, 6 out]
                    n604 = invoke on="控件配置文件" class="Tbl (严格)" method="Set Cell Value"("X Index"=0 ("X索引"), "Y Index"=w755, "Value"=w756) -> ()  [unwired: 3 in, 6 out]
                  }
                  frame "关联到曲线3" {
                    w766 = T9 32 items=["刷新间隔", "波特率", "布尔1设置项", "布尔2设置项", "布尔3设置项", "布尔4设置项", "布尔5设置项", "布尔6设置项", "布尔7设置项", "布尔8设置项", "显控1设置", "显控2设置", "显控3设置", "显控4设置", "显控5设置", "显控6设置", "显控7设置", "显控8设置", "显控9设置", "显控10设置", "显控11设置", "显控12设置", "设控1设置", "设控2设置", "设控3设置", "设控4设置", "设控5设置", "设控6设置", "设控7设置", "设控8设置", "曲线1设置", "曲线2设置", "曲线3设置", "曲线4设置", "曲线5设置", "曲线6设置", "曲线7设置", "曲线8设置", "曲线9设置", "曲线10设置", "曲线11设置", "曲线12设置", "曲线13设置", "曲线14设置", "曲线15设置", "曲线16设置", "曲线17设置", "曲线18设置", "曲线19设置", "曲线20设置", "曲线21设置", "曲线22设置", "曲线23设置", "曲线24设置", "曲线25设置", "曲线26设置", "曲线27设置", "曲线28设置", "曲线29设置", "曲线30设置", "曲线31设置", "曲线32设置", "曲线33设置", "曲线34设置", "曲线35设置", "曲线36设置", "曲线37设置", "曲线38设置", "曲线39设置", "曲线40设置", "曲线41设置", "曲线42设置", "曲线43设置", "曲线44设置", "曲线45设置", "曲线46设置", "曲线47设置", "曲线48设置", "曲线49设置", "曲线50设置", "曲线51设置", "曲线52设置", "曲线53设置", "曲线54设置", "曲线55设置", "曲线56设置", "曲线57设置", "曲线58设置", "曲线59设置", "曲线60设置", "曲线61设置", "曲线62设置", "曲线63设置", "曲线64设置", "ID值", "数据模式"] ("DataInitDef")
                    n605 = property on="表格" class="Tbl (严格)"() -> ("Selection Start"=w775:T1)  [unwired: 2 in, 2 out]
                    n606 = Unbundle By Name(w775) -> ("Row"=w773:i32)
                    n607 = property on="表格" class="Tbl (严格)"() -> ("Value"=w774:string[][])  [unwired: 2 in, 2 out]
                    n608 = Number To Decimal String(number=w773) -> (decimal integer string=w770:string)  [unwired: 1 in]
                    n609 = Index Array(array=w774, index (row)=w773, index (col)=0 ("禁用的索引 (列)")) -> (element=w768:string)
                    n610 = String Subset(string=w768, length (rest)=16 ("长度（剩余）")) -> (substring=w767:string)  [unwired: 1 in]
                    n611 = property on="曲线3设置" class="Str"("Val(Sgnl)"=w767) -> ()  [unwired: 2 in, 2 out]
                    n612 = invoke on="控件配置文件" class="Tbl (严格)" method="Set Cell Value"("X Index"=1 ("X索引"), "Y Index"=w766, "Value"=w770) -> ()  [unwired: 3 in, 6 out]
                    n613 = invoke on="控件配置文件" class="Tbl (严格)" method="Set Cell Value"("X Index"=0 ("X索引"), "Y Index"=w766, "Value"=w767) -> ()  [unwired: 3 in, 6 out]
                  }
                  frame "关联到曲线4" {
                    w777 = T9 33 items=["刷新间隔", "波特率", "布尔1设置项", "布尔2设置项", "布尔3设置项", "布尔4设置项", "布尔5设置项", "布尔6设置项", "布尔7设置项", "布尔8设置项", "显控1设置", "显控2设置", "显控3设置", "显控4设置", "显控5设置", "显控6设置", "显控7设置", "显控8设置", "显控9设置", "显控10设置", "显控11设置", "显控12设置", "设控1设置", "设控2设置", "设控3设置", "设控4设置", "设控5设置", "设控6设置", "设控7设置", "设控8设置", "曲线1设置", "曲线2设置", "曲线3设置", "曲线4设置", "曲线5设置", "曲线6设置", "曲线7设置", "曲线8设置", "曲线9设置", "曲线10设置", "曲线11设置", "曲线12设置", "曲线13设置", "曲线14设置", "曲线15设置", "曲线16设置", "曲线17设置", "曲线18设置", "曲线19设置", "曲线20设置", "曲线21设置", "曲线22设置", "曲线23设置", "曲线24设置", "曲线25设置", "曲线26设置", "曲线27设置", "曲线28设置", "曲线29设置", "曲线30设置", "曲线31设置", "曲线32设置", "曲线33设置", "曲线34设置", "曲线35设置", "曲线36设置", "曲线37设置", "曲线38设置", "曲线39设置", "曲线40设置", "曲线41设置", "曲线42设置", "曲线43设置", "曲线44设置", "曲线45设置", "曲线46设置", "曲线47设置", "曲线48设置", "曲线49设置", "曲线50设置", "曲线51设置", "曲线52设置", "曲线53设置", "曲线54设置", "曲线55设置", "曲线56设置", "曲线57设置", "曲线58设置", "曲线59设置", "曲线60设置", "曲线61设置", "曲线62设置", "曲线63设置", "曲线64设置", "ID值", "数据模式"] ("DataInitDef")
                    n614 = property on="表格" class="Tbl (严格)"() -> ("Selection Start"=w786:T1)  [unwired: 2 in, 2 out]
                    n615 = Unbundle By Name(w786) -> ("Row"=w784:i32)
                    n616 = property on="表格" class="Tbl (严格)"() -> ("Value"=w785:string[][])  [unwired: 2 in, 2 out]
                    n617 = Number To Decimal String(number=w784) -> (decimal integer string=w781:string)  [unwired: 1 in]
                    n618 = Index Array(array=w785, index (row)=w784, index (col)=0 ("禁用的索引 (列)")) -> (element=w779:string)
                    n619 = String Subset(string=w779, length (rest)=16 ("长度（剩余）")) -> (substring=w778:string)  [unwired: 1 in]
                    n620 = property on="曲线4设置" class="Str"("Val(Sgnl)"=w778) -> ()  [unwired: 2 in, 2 out]
                    n621 = invoke on="控件配置文件" class="Tbl (严格)" method="Set Cell Value"("X Index"=1 ("X索引"), "Y Index"=w777, "Value"=w781) -> ()  [unwired: 3 in, 6 out]
                    n622 = invoke on="控件配置文件" class="Tbl (严格)" method="Set Cell Value"("X Index"=0 ("X索引"), "Y Index"=w777, "Value"=w778) -> ()  [unwired: 3 in, 6 out]
                  }
                  frame "关联到曲线5" {
                    w788 = T9 34 items=["刷新间隔", "波特率", "布尔1设置项", "布尔2设置项", "布尔3设置项", "布尔4设置项", "布尔5设置项", "布尔6设置项", "布尔7设置项", "布尔8设置项", "显控1设置", "显控2设置", "显控3设置", "显控4设置", "显控5设置", "显控6设置", "显控7设置", "显控8设置", "显控9设置", "显控10设置", "显控11设置", "显控12设置", "设控1设置", "设控2设置", "设控3设置", "设控4设置", "设控5设置", "设控6设置", "设控7设置", "设控8设置", "曲线1设置", "曲线2设置", "曲线3设置", "曲线4设置", "曲线5设置", "曲线6设置", "曲线7设置", "曲线8设置", "曲线9设置", "曲线10设置", "曲线11设置", "曲线12设置", "曲线13设置", "曲线14设置", "曲线15设置", "曲线16设置", "曲线17设置", "曲线18设置", "曲线19设置", "曲线20设置", "曲线21设置", "曲线22设置", "曲线23设置", "曲线24设置", "曲线25设置", "曲线26设置", "曲线27设置", "曲线28设置", "曲线29设置", "曲线30设置", "曲线31设置", "曲线32设置", "曲线33设置", "曲线34设置", "曲线35设置", "曲线36设置", "曲线37设置", "曲线38设置", "曲线39设置", "曲线40设置", "曲线41设置", "曲线42设置", "曲线43设置", "曲线44设置", "曲线45设置", "曲线46设置", "曲线47设置", "曲线48设置", "曲线49设置", "曲线50设置", "曲线51设置", "曲线52设置", "曲线53设置", "曲线54设置", "曲线55设置", "曲线56设置", "曲线57设置", "曲线58设置", "曲线59设置", "曲线60设置", "曲线61设置", "曲线62设置", "曲线63设置", "曲线64设置", "ID值", "数据模式"] ("DataInitDef")
                    n623 = property on="表格" class="Tbl (严格)"() -> ("Selection Start"=w797:T1)  [unwired: 2 in, 2 out]
                    n624 = Unbundle By Name(w797) -> ("Row"=w795:i32)
                    n625 = property on="表格" class="Tbl (严格)"() -> ("Value"=w796:string[][])  [unwired: 2 in, 2 out]
                    n626 = Number To Decimal String(number=w795) -> (decimal integer string=w792:string)  [unwired: 1 in]
                    n627 = Index Array(array=w796, index (row)=w795, index (col)=0 ("禁用的索引 (列)")) -> (element=w790:string)
                    n628 = String Subset(string=w790, length (rest)=16 ("长度（剩余）")) -> (substring=w789:string)  [unwired: 1 in]
                    n629 = property on="曲线5设置" class="Str"("Val(Sgnl)"=w789) -> ()  [unwired: 2 in, 2 out]
                    n630 = invoke on="控件配置文件" class="Tbl (严格)" method="Set Cell Value"("X Index"=1 ("X索引"), "Y Index"=w788, "Value"=w792) -> ()  [unwired: 3 in, 6 out]
                    n631 = invoke on="控件配置文件" class="Tbl (严格)" method="Set Cell Value"("X Index"=0 ("X索引"), "Y Index"=w788, "Value"=w789) -> ()  [unwired: 3 in, 6 out]
                  }
                  frame "关联到曲线6" {
                    w799 = T9 35 items=["刷新间隔", "波特率", "布尔1设置项", "布尔2设置项", "布尔3设置项", "布尔4设置项", "布尔5设置项", "布尔6设置项", "布尔7设置项", "布尔8设置项", "显控1设置", "显控2设置", "显控3设置", "显控4设置", "显控5设置", "显控6设置", "显控7设置", "显控8设置", "显控9设置", "显控10设置", "显控11设置", "显控12设置", "设控1设置", "设控2设置", "设控3设置", "设控4设置", "设控5设置", "设控6设置", "设控7设置", "设控8设置", "曲线1设置", "曲线2设置", "曲线3设置", "曲线4设置", "曲线5设置", "曲线6设置", "曲线7设置", "曲线8设置", "曲线9设置", "曲线10设置", "曲线11设置", "曲线12设置", "曲线13设置", "曲线14设置", "曲线15设置", "曲线16设置", "曲线17设置", "曲线18设置", "曲线19设置", "曲线20设置", "曲线21设置", "曲线22设置", "曲线23设置", "曲线24设置", "曲线25设置", "曲线26设置", "曲线27设置", "曲线28设置", "曲线29设置", "曲线30设置", "曲线31设置", "曲线32设置", "曲线33设置", "曲线34设置", "曲线35设置", "曲线36设置", "曲线37设置", "曲线38设置", "曲线39设置", "曲线40设置", "曲线41设置", "曲线42设置", "曲线43设置", "曲线44设置", "曲线45设置", "曲线46设置", "曲线47设置", "曲线48设置", "曲线49设置", "曲线50设置", "曲线51设置", "曲线52设置", "曲线53设置", "曲线54设置", "曲线55设置", "曲线56设置", "曲线57设置", "曲线58设置", "曲线59设置", "曲线60设置", "曲线61设置", "曲线62设置", "曲线63设置", "曲线64设置", "ID值", "数据模式"] ("DataInitDef")
                    n632 = property on="表格" class="Tbl (严格)"() -> ("Selection Start"=w808:T1)  [unwired: 2 in, 2 out]
                    n633 = Unbundle By Name(w808) -> ("Row"=w806:i32)
                    n634 = property on="表格" class="Tbl (严格)"() -> ("Value"=w807:string[][])  [unwired: 2 in, 2 out]
                    n635 = Number To Decimal String(number=w806) -> (decimal integer string=w803:string)  [unwired: 1 in]
                    n636 = Index Array(array=w807, index (row)=w806, index (col)=0 ("禁用的索引 (列)")) -> (element=w801:string)
                    n637 = String Subset(string=w801, length (rest)=16 ("长度（剩余）")) -> (substring=w800:string)  [unwired: 1 in]
                    n638 = property on="曲线6设置" class="Str"("Val(Sgnl)"=w800) -> ()  [unwired: 2 in, 2 out]
                    n639 = invoke on="控件配置文件" class="Tbl (严格)" method="Set Cell Value"("X Index"=1 ("X索引"), "Y Index"=w799, "Value"=w803) -> ()  [unwired: 3 in, 6 out]
                    n640 = invoke on="控件配置文件" class="Tbl (严格)" method="Set Cell Value"("X Index"=0 ("X索引"), "Y Index"=w799, "Value"=w800) -> ()  [unwired: 3 in, 6 out]
                  }
                  frame "关联到曲线7" {
                    w810 = T9 36 items=["刷新间隔", "波特率", "布尔1设置项", "布尔2设置项", "布尔3设置项", "布尔4设置项", "布尔5设置项", "布尔6设置项", "布尔7设置项", "布尔8设置项", "显控1设置", "显控2设置", "显控3设置", "显控4设置", "显控5设置", "显控6设置", "显控7设置", "显控8设置", "显控9设置", "显控10设置", "显控11设置", "显控12设置", "设控1设置", "设控2设置", "设控3设置", "设控4设置", "设控5设置", "设控6设置", "设控7设置", "设控8设置", "曲线1设置", "曲线2设置", "曲线3设置", "曲线4设置", "曲线5设置", "曲线6设置", "曲线7设置", "曲线8设置", "曲线9设置", "曲线10设置", "曲线11设置", "曲线12设置", "曲线13设置", "曲线14设置", "曲线15设置", "曲线16设置", "曲线17设置", "曲线18设置", "曲线19设置", "曲线20设置", "曲线21设置", "曲线22设置", "曲线23设置", "曲线24设置", "曲线25设置", "曲线26设置", "曲线27设置", "曲线28设置", "曲线29设置", "曲线30设置", "曲线31设置", "曲线32设置", "曲线33设置", "曲线34设置", "曲线35设置", "曲线36设置", "曲线37设置", "曲线38设置", "曲线39设置", "曲线40设置", "曲线41设置", "曲线42设置", "曲线43设置", "曲线44设置", "曲线45设置", "曲线46设置", "曲线47设置", "曲线48设置", "曲线49设置", "曲线50设置", "曲线51设置", "曲线52设置", "曲线53设置", "曲线54设置", "曲线55设置", "曲线56设置", "曲线57设置", "曲线58设置", "曲线59设置", "曲线60设置", "曲线61设置", "曲线62设置", "曲线63设置", "曲线64设置", "ID值", "数据模式"] ("DataInitDef")
                    n641 = property on="表格" class="Tbl (严格)"() -> ("Selection Start"=w819:T1)  [unwired: 2 in, 2 out]
                    n642 = Unbundle By Name(w819) -> ("Row"=w817:i32)
                    n643 = property on="表格" class="Tbl (严格)"() -> ("Value"=w818:string[][])  [unwired: 2 in, 2 out]
                    n644 = Number To Decimal String(number=w817) -> (decimal integer string=w814:string)  [unwired: 1 in]
                    n645 = Index Array(array=w818, index (row)=w817, index (col)=0 ("禁用的索引 (列)")) -> (element=w812:string)
                    n646 = String Subset(string=w812, length (rest)=16 ("长度（剩余）")) -> (substring=w811:string)  [unwired: 1 in]
                    n647 = property on="曲线7设置" class="Str"("Val(Sgnl)"=w811) -> ()  [unwired: 2 in, 2 out]
                    n648 = invoke on="控件配置文件" class="Tbl (严格)" method="Set Cell Value"("X Index"=1 ("X索引"), "Y Index"=w810, "Value"=w814) -> ()  [unwired: 3 in, 6 out]
                    n649 = invoke on="控件配置文件" class="Tbl (严格)" method="Set Cell Value"("X Index"=0 ("X索引"), "Y Index"=w810, "Value"=w811) -> ()  [unwired: 3 in, 6 out]
                  }
                  frame "关联到曲线8" {
